vi "GCode Parser - SoftMotion Example.vi"() -> ()   [LabVIEW 2014]
uses:
  Typedefs/Motion Parameters.ctl
  <vilib>/Motion/Express/_s/nimc.fb.straightLineMove.blendMode.ctl
  GCode Parser/GCode Command Cluster.ctl
  <vilib>/Motion/Express/_s/nimc.ex.clearFaults.clearFaults.axis.vi
  <vilib>/Motion/Express/_s/nimc.ex.power.power.axis.vi
  <vilib>/Motion/Express/_s/nimc.ex.resetPosition.resetPosition.axis.vi
  <vilib>/Motion/Express/_s/nimc.ex.straightLineMove.startStraightLineMove.coordinate.modeAbsolute.blendEnable.1.vi
  <vilib>/Motion/Express/_s/nimc.ex.arcMove.startArcMove.coordinate.modeCircular.blendEnable.1.vi
  <vilib>/Motion/Express/_s/nimc.ex.stopMove.stop.coordinate.modeDecelerate.vi
  <vilib>/Motion/Express/_s/nimc.ex.read.readTrajectoryData.coordinate.vi
  <vilib>/Motion/Express/_s/nimc.ex.read.readExecutionData.axis.vi
  <vilib>/Motion/BlockNode/FB.NIMotion.xnode
  <vilib>/Motion/Express/_s/nimc.fb.arcMove.blendMode.ctl
panel:
  out "Current GCode Command":T1
  in  "Motion Parameters":T2={"timeout"=-1.0, "acceleration"=10000.0, "deceleration"=10000.0, "accel. jerk"=100000.0, "decel. jerk"=100000.0, "blend mode"=10551334, "blend delay"=-1.0, "smoothing"=0.5, "last blend"=FALSE} {"blend mode" items=["At Profile Complete"=10551335, "At Deceleration"=10551334, "After Delay"=10551336]}
  in  "G0 Velocity":dbl=20.0
  in  "Position Scale":dbl=1.0
  in  "Velocity Scale":dbl=1.0
  out "Global Stop":bool
  out "text":string
  in  "Quit":bool
  out "Iterations":i32
  out "Command Array":T1[](array[typedef])
  out "error out":errorcluster
  out "Position Plot":cluster{dbl[], dbl[]}(graph)
  out "Axis Positions":T4(graph)
  out "Axis Velocities":T5(graph)
  in  "start index":i32
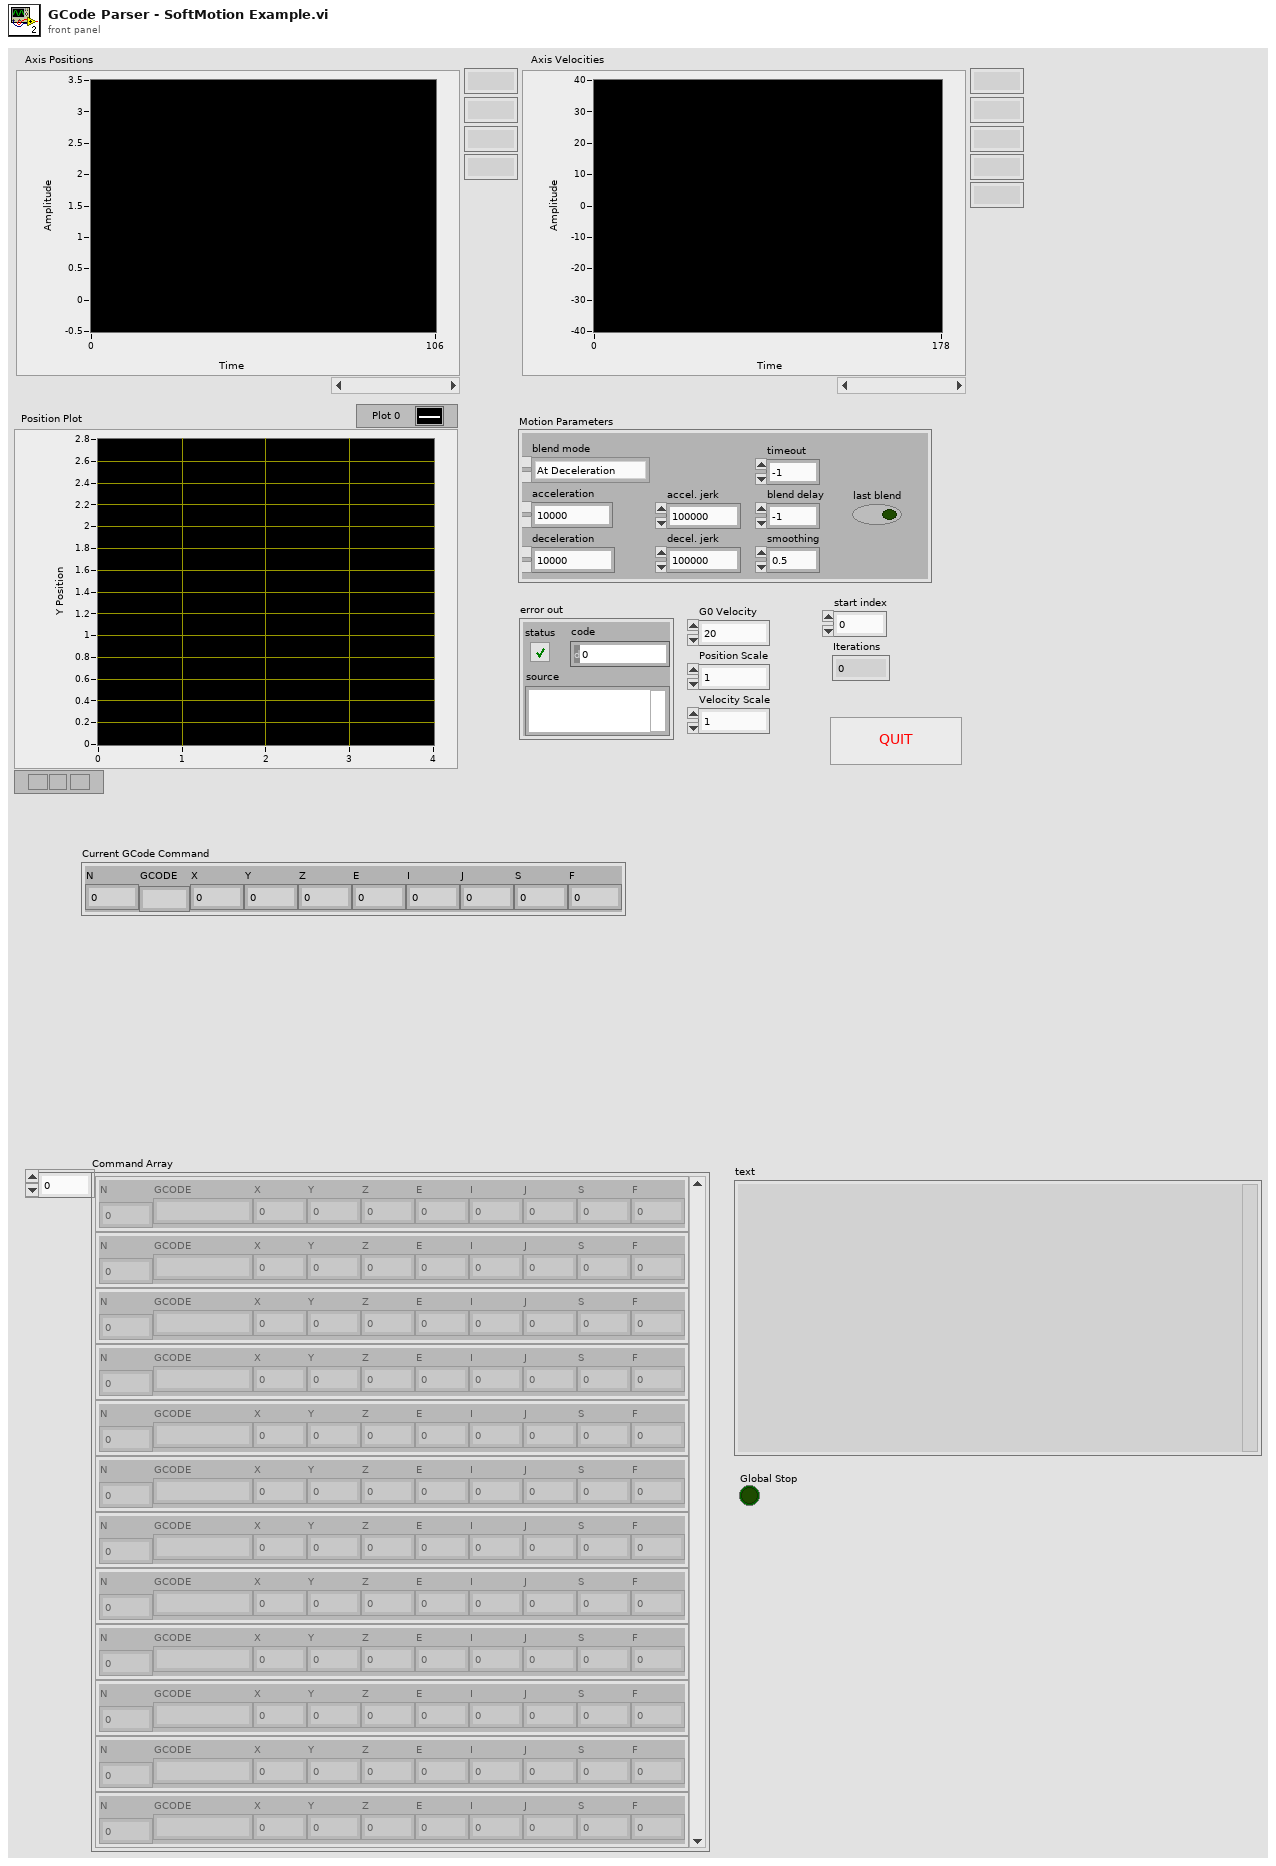
[diagram p1: front panel]
types:
  T1 = typedef "GCode Command Cluster.ctl" = cluster{"N":dbl, "GCODE":string, "X":dbl, "Y":dbl, "Z":dbl, "E":dbl, "I":dbl, "J":dbl, "S":dbl, "F":dbl}
  T2 = typedef "Motion Parameters.ctl" = cluster{"timeout":dbl, "acceleration":dbl, "deceleration":dbl, "accel. jerk":dbl, "decel. jerk":dbl, "blend mode":T3, "blend delay":dbl, "smoothing":dbl, "last blend":bool}
  T3 = typedef "nimc.fb.straightLineMove.blendMode.ctl" = i32
  T4 = cluster{"commanded pos.[] out[0]":dbl, "commanded pos.[] out[1]":dbl, "commanded pos.[] out[2]":dbl, "commanded pos.[] out[3]":dbl}
  T5 = cluster{"commanded vel.":dbl, "velocity":dbl, "velocity":dbl, "velocity":dbl, "velocity":dbl}
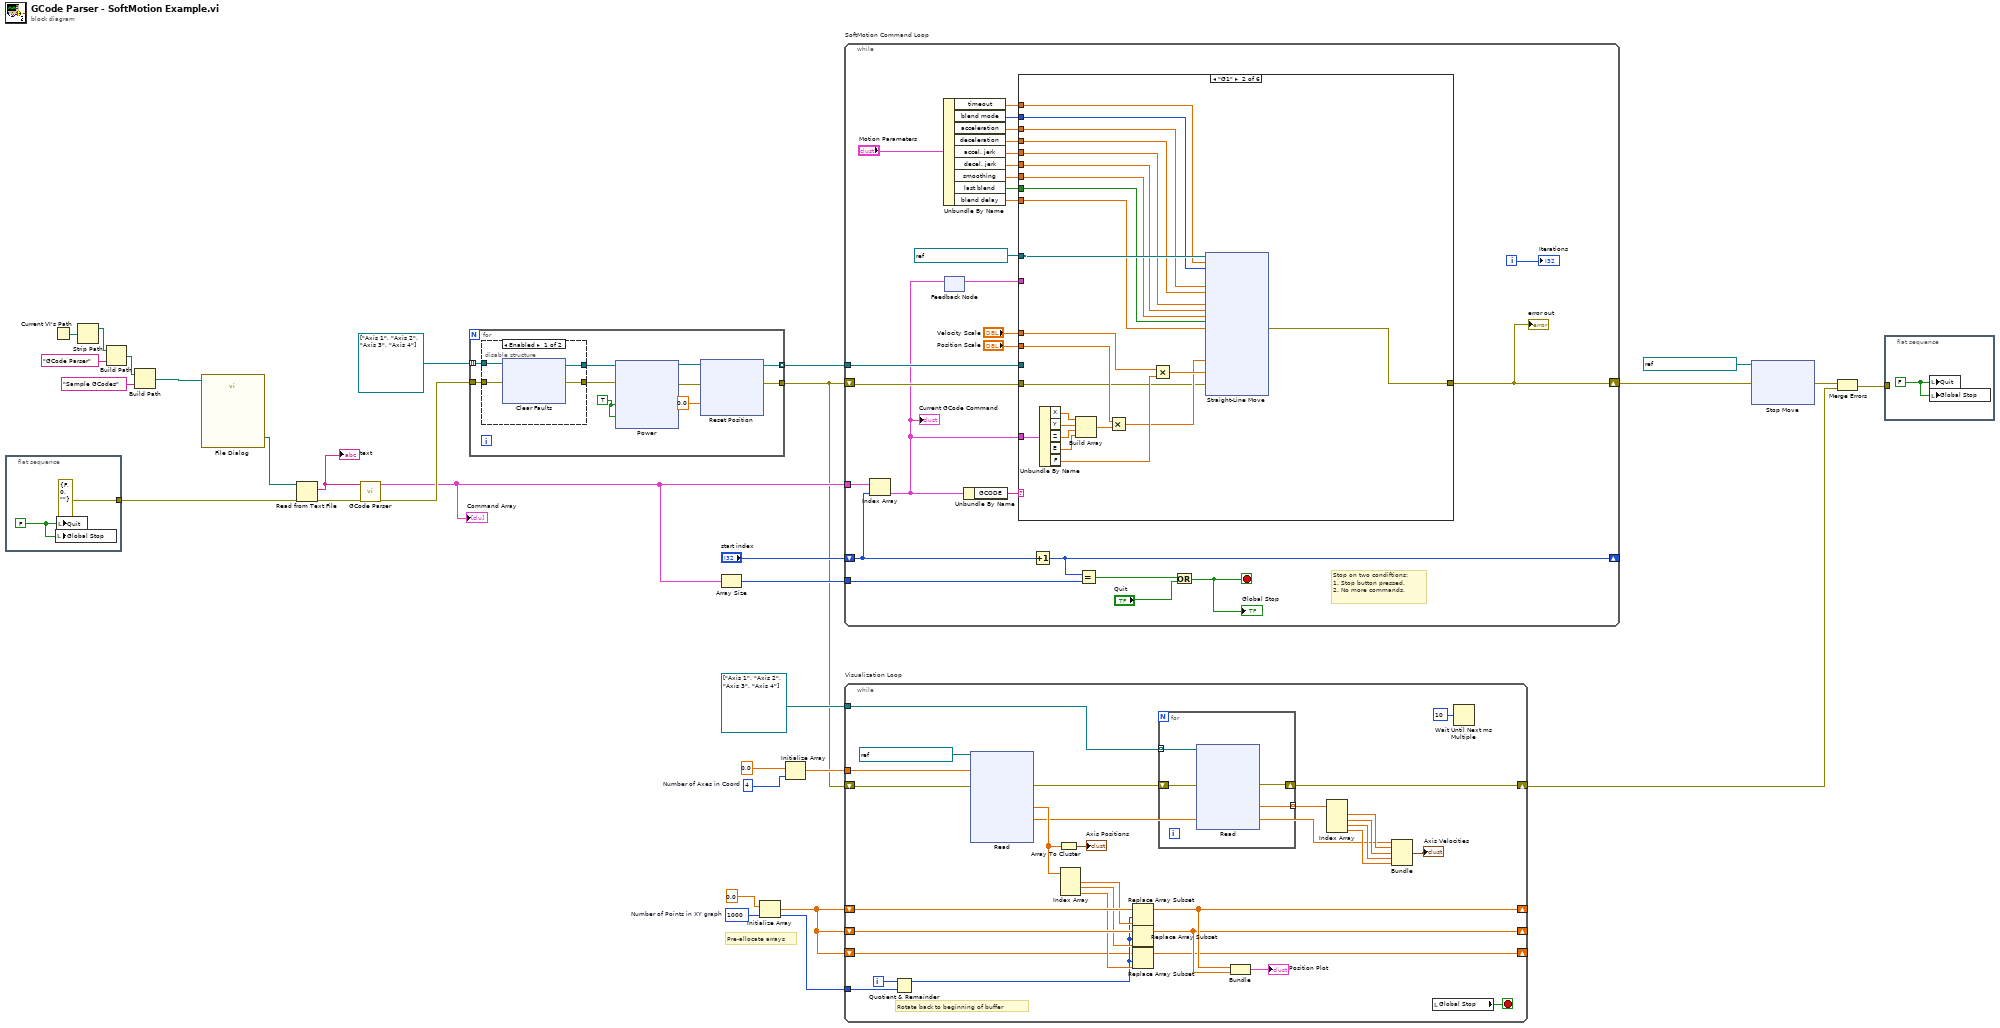
[diagram p0: block diagram]
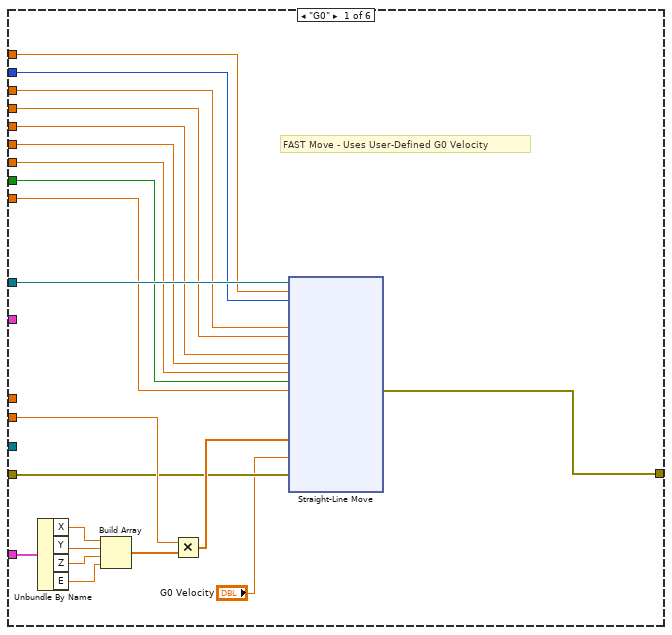
[diagram p2: hidden frame]
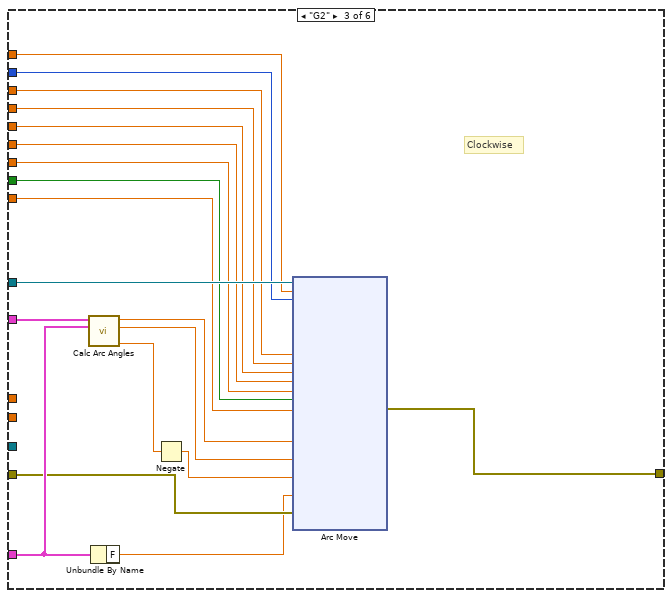
[diagram p3: hidden frame]
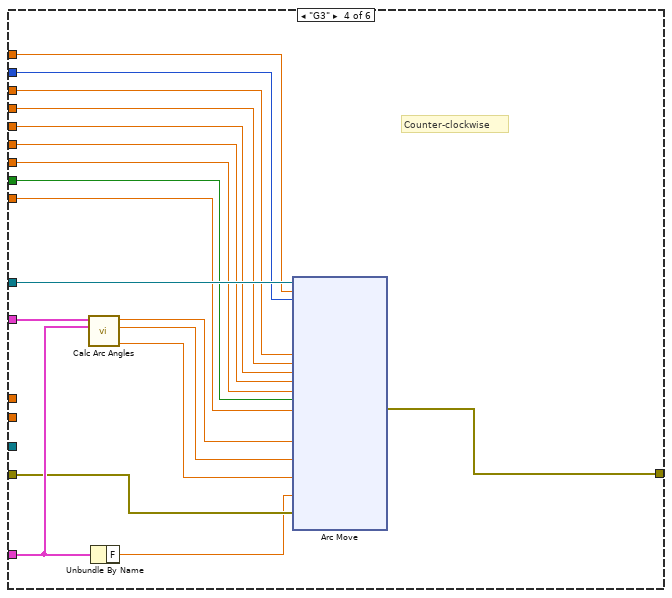
[diagram p4: hidden frame]
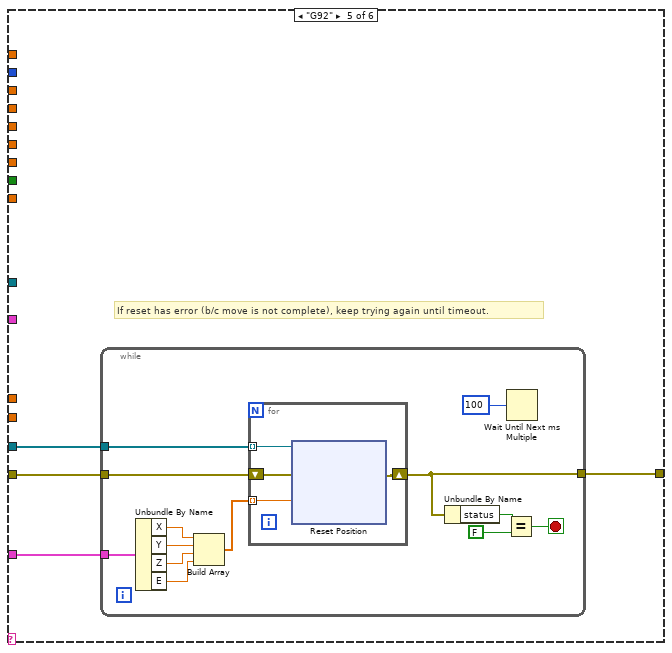
[diagram p5: hidden frame]
diagram:
  w25 = 1000  # Number of Points in XY graph
  w27 = 4  # Number of Axes in Coord
  # "Pre-allocate arrays"
  n1 = flat-sequence {
    tunnel: [errorcluster {"status"=FALSE, "code"=0, "source"=""} ("error out")] -> w20
    frame #0 {
      w30 = FALSE ("Example Done")
      n2 = local write "Global Stop"(w30) -> ()
      n3 = local write "Quit"(w30) -> ()
    }
  }
  n4 = Current VI's Path() -> (path=w7:path)
  n5 = Strip Path(path=w7) -> (stripped path=w6:path)  [unwired: 1 out]
  n6 = Build Path(base path=w6, name or relative path="GCode Parser") -> (appended path=w2:path)
  n7 = Build Path(base path=w2, name or relative path="Sample GCodes") -> (appended path=w1:path)
  n8 = call "File Dialog"("start path"=w1) -> ("selected path"=w4:path)  [unwired: 11 in, 3 out]
  n9 = Read from Text File(file (use dialog)=w4, error in=w20) -> (text=w22:string, error out=w21:errorcluster)  [unwired: 2 in, 2 out]
  "text" <- w22
  n10 = call "GCode Parser.vi"("error in (no error)"=w21, "String in"=w22) -> ("error out"=w19:errorcluster, "Command Array"=w15:T1[])  [unwired: 8 in]
  "Command Array" <- w15
  n11 = for {
    tunnel: refnum<k21>[] ["Axis 1", "Axis 2", "Axis 3", "Axis 4"] -> [w41] mode=indexing
    tunnel: w19 -> [w40]
    tunnel: [w39] -> w12
    tunnel: [w32] -> w16 mode=indexing
    w34 = TRUE ("enable axis")
    n12 = disable-structure shown="Enabled" {
      disable-tunnel: w41 -> [w45 w51]
      disable-tunnel: w40 -> [w44 w50]
      disable-tunnel: [w43 w51] -> w37
      disable-tunnel: [w42 w50] -> w35
      frame Enabled {
        n13 = xnode ("Clear Faults")("resource"=w45, "error in"=w44) -> ("resource out"=w43:refnum<k21>, "error out"=w42:errorcluster)
      }
      frame Disabled {
      }
    }
    n14 = xnode ("Power")("enable axis"=w34, "enable drive"=w34, "resource"=w37, "error in"=w35) -> ("resource out"=w36:refnum<k21>, "error out"=w33:errorcluster)
    n15 = xnode ("Reset Position")("position"=0.0, "resource"=w36, "error in"=w33) -> ("resource out"=w32:refnum<k21>, "error out"=w39:errorcluster)
  }
  n16 = Array Size(array=w15) -> (size(s)=w14:i32)
  n17 = Initialize Array(0.0 ("element"), w25) -> (w24:dbl[])
  n18 = Initialize Array(0.0 ("element"), w27) -> (w23:dbl[])
  n19 = while "SoftMotion Command Loop" {
    tunnel: w15 -> [w86]
    shift-right: [w83] -> _
    shift-left: "start index" -> [w85]
    shift-right: [w90] -> w9
    shift-left: w12 -> [w89]
    tunnel: w16 -> [w88]
    tunnel: w14 -> [w84]
    i -> [w87]
    stop <- w81 stop-if-true
    # "Stop on two condiftions:\n1. Stop button pressed.\n2. No more commands."
    n20 = Index Array(array=w86, index=w85) -> (element=w68:T1)
    "Current GCode Command" <- w68
    n21 = Unbundle By Name("Motion Parameters") -> ("timeout"=w77:dbl, "blend mode"=w76:T3, "acceleration"=w75:dbl, "deceleration"=w74:dbl, "accel. jerk"=w73:dbl, "decel. jerk"=w72:dbl, "smoothing"=w70:dbl, "last blend"=w71:bool, "blend delay"=w69:dbl)
    n22 = feedback-in #1(w68) -> ()
    n23 = feedback #1() -> (w67:T1)  [unwired: 1 in]
    n24 = Unbundle By Name(w68) -> ("GCODE"=w93:string)
    n25 = case shown="\"G1\"" w93 {
      tunnel: refnum<k21> "Coordinate Space 1" ("Motion Resource") -> [w106 w147 w196 w236 _ _]
      tunnel: [w114 w157 w186 w226 w259 w285] -> w90
      tunnel: "Velocity Scale" -> [_ w135 _ _ _ _]
      tunnel: w68 -> [w109 w151 w193 w233 w260 _]
      tunnel: "Position Scale" -> [w107 w148 _ _ _ _]
      tunnel: w89 -> [w104 w145 w187 w227 w261 w285]
      tunnel: w77 -> [w103 w144 w192 w232 _ _]
      tunnel: w76 -> [w102 w143 w178 w220 _ _]
      tunnel: w75 -> [w101 w142 w191 w231 _ _]
      tunnel: w74 -> [w100 w141 w190 w230 _ _]
      tunnel: w73 -> [w99 w140 w189 w229 _ _]
      tunnel: w72 -> [w98 w139 w188 w228 _ _]
      tunnel: w70 -> [w97 w138 w179 w221 _ _]
      tunnel: w71 -> [w96 w137 w180 w222 _ _]
      tunnel: w69 -> [w95 w136 w181 w223 _ _]
      tunnel: w88 -> [_ _ _ _ w262 _]
      tunnel: w67 -> [_ _ w195 w235 _ _]
      frame "G0" {
        # "FAST Move - Uses User-Defined G0 Velocity"
        n26 = Unbundle By Name(w109) -> ("X"=w113:dbl, "Y"=w112:dbl, "Z"=w111:dbl, "E"=w110:dbl)
        n27 = Build Array(w113, w112, w111, w110) -> (w108:dbl[])
        n28 = Multiply(x=w107, y=w108) -> (x*y=w105:dbl[])
        n29 = xnode ("Straight-Line Move")("position[]"=w105, "velocity"="G0 Velocity", "error in"=w104, "resource"=w106, "timeout"=w103, "blend mode"=w102, "acceleration"=w101, "deceleration"=w100, "accel. jerk"=w99, "decel. jerk"=w98, "smoothing"=w97, "last blend"=w96, "blend delay"=w95) -> ("error out"=w114:errorcluster)  [unwired: 2 out]
      }
      frame "G1" {
        n30 = Unbundle By Name(w151) -> ("X"=w156:dbl, "Y"=w155:dbl, "Z"=w154:dbl, "E"=w153:dbl, "F"=w152:dbl)
        n31 = Build Array(w156, w155, w154, w153) -> (w149:dbl[])
        n32 = Multiply(x=w148, y=w149) -> (x*y=w146:dbl[])
        n33 = Multiply(x=w135, y=w152) -> (x*y=w150:dbl)
        n34 = xnode ("Straight-Line Move")("position[]"=w146, "velocity"=w150, "error in"=w145, "resource"=w147, "timeout"=w144, "blend mode"=w143, "acceleration"=w142, "deceleration"=w141, "accel. jerk"=w140, "decel. jerk"=w139, "smoothing"=w138, "last blend"=w137, "blend delay"=w136) -> ("error out"=w157:errorcluster)  [unwired: 2 out]
      }
      frame "G2" {
        # "Clockwise"
        n35 = call "Calc Arc Angles.vi"("Arc CMD"=w193, "Initial CMD"=w195) -> ("travel angle out"=w184:dbl, "start angle (tangent)"=w183:dbl, "R"=w194:dbl)  [unwired: 7 in]
        n36 = Unbundle By Name(w193) -> ("F"=w182:dbl)
        n37 = Negate(x=w184) -> (-x=w185:dbl)
        n38 = xnode ("Arc Move")("radius"=w194, "start angle"=w183, "travel angle"=w185, "velocity"=w182, "error in"=w187, "resource"=w196, "timeout"=w192, "blend mode"=w178, "acceleration"=w191, "deceleration"=w190, "accel. jerk"=w189, "decel. jerk"=w188, "smoothing"=w179, "last blend"=w180, "blend delay"=w181) -> ("error out"=w186:errorcluster)  [unwired: 2 out]
      }
      frame "G3" {
        # "Counter-clockwise"
        n39 = call "Calc Arc Angles.vi"("Arc CMD"=w233, "Initial CMD"=w235) -> ("travel angle out"=w219:dbl, "start angle (tangent)"=w225:dbl, "R"=w234:dbl)  [unwired: 7 in]
        n40 = Unbundle By Name(w233) -> ("F"=w224:dbl)
        n41 = xnode ("Arc Move")("radius"=w234, "start angle"=w225, "travel angle"=w219, "velocity"=w224, "error in"=w227, "resource"=w236, "timeout"=w232, "blend mode"=w220, "acceleration"=w231, "deceleration"=w230, "accel. jerk"=w229, "decel. jerk"=w228, "smoothing"=w221, "last blend"=w222, "blend delay"=w223) -> ("error out"=w226:errorcluster)  [unwired: 2 out]
      }
      frame "G92" {
        # "If reset has error (b/c move is not complete), keep trying again until timeout."
        n42 = while {
          tunnel: [w272] -> w259
          tunnel: w262 -> [w270]
          tunnel: w261 -> [w269]
          tunnel: w260 -> [w264]
          stop <- w271 stop-if-true
          n43 = Unbundle By Name(w264) -> ("X"=w268:dbl, "Y"=w267:dbl, "Z"=w266:dbl, "E"=w265:dbl)
          n44 = Build Array(w268, w267, w266, w265) -> (w263:dbl[])
          n45 = for {
            tunnel: w270 -> [w278] mode=indexing
            shift-right: [w279] -> w272
            shift-left: w269 -> [w277]
            tunnel: w263 -> [w276] mode=indexing
            n46 = xnode ("Reset Position")("position"=w276, "resource"=w278, "error in"=w277) -> ("error out"=w279:errorcluster)  [unwired: 1 out]
          }
          n47 = Unbundle By Name(w272) -> ("status"=w274:bool)
          n48 = Equal?(x=w274, y=FALSE) -> (x = y?=w271:bool)
          n49 = Wait Until Next ms Multiple(millisecond multiple=u32 100) -> ()  [unwired: 1 out]
        }
      }
      frame Default {
        # "Empty case for all other codes."
      }
    }
    "error out" <- w90
    n50 = Increment(x=w85) -> (x+1=w83:i32)
    n51 = Equal?(x=w83, y=w84) -> (x = y?=w82:bool)
    n52 = Or(x=w82, y="Quit") -> (x .or. y?=w81:bool)
    "Global Stop" <- w81
    "Iterations" <- w87
  }
  n53 = while "Visualization Loop" {
    shift-right: [w304] -> _
    shift-left: w24 -> [w314]
    shift-right: [w286] -> w11
    shift-left: w12 -> [w294]
    shift-right: [w303] -> _
    shift-left: w24 -> [w312]
    tunnel: w25 -> [w309]
    shift-right: [w302] -> _
    shift-left: w24 -> [w305]
    tunnel: w23 -> [w291]
    tunnel: refnum<k21>[] ["Axis 1", "Axis 2", "Axis 3", "Axis 4"] -> [w300]
    i -> [w308]
    stop <- w288 stop-if-true
    # "Rotate back to beginning of buffer"
    n54 = Quotient & Remainder(x=w308, y=w309) -> (x-y*floor(x/y)=w306:i32)  [unwired: 1 out]
    n55 = xnode ("Read")("resource"=refnum<k21> "Coordinate Space 1" ("Motion Resource"), "commanded pos.[]"=w291, "error in"=w294) -> ("commanded pos.[] out"=w292:dbl[], "commanded vel."=w289:dbl, "error out"=w293:errorcluster)  [unwired: 3 out]
    n56 = Array To Cluster(array=w292) -> (cluster=→"Axis Positions":T4)
    n57 = Index Array(array=w292) -> (element #1=w313:dbl, element #2=w311:dbl, element #3=w307:dbl)  [unwired: 3 in]
    n58 = Replace Array Subset(array=w314, new element=w313, index=w306) -> (w304:dbl[])
    n59 = Replace Array Subset(array=w312, new element=w311, index=w306) -> (w303:dbl[])
    n60 = Replace Array Subset(array=w305, new element=w307, index=w306) -> (w302:dbl[])
    n61 = for {
      tunnel: w300 -> [w328] mode=indexing
      tunnel: [w327] -> w299 mode=indexing
      shift-right: [w325] -> w286
      shift-left: w293 -> [w326]
      n62 = xnode ("Read")("resource"=w328, "error in"=w326) -> ("velocity"=w327:dbl, "error out"=w325:errorcluster)  [unwired: 5 out]
    }
    n63 = Bundle(w304, w303) -> (→"Position Plot":cluster{dbl[], dbl[]})  [unwired: 1 in]
    n64 = Index Array(array=w299) -> (element #1=w298:dbl, element #2=w297:dbl, element #3=w296:dbl, element #4=w290:dbl)  [unwired: 4 in]
    n65 = Bundle("commanded vel."=w289, "velocity"=w298, "velocity"=w297, "velocity"=w296, "velocity"=w290) -> (→"Axis Velocities":T5)  [unwired: 1 in]
    n66 = local read "Global Stop"() -> (w288:bool)
    n67 = Wait Until Next ms Multiple(millisecond multiple=u32 10) -> ()  [unwired: 1 out]
  }
  n68 = xnode ("Stop Move")("resource"=refnum<k21> "Coordinate Space 1" ("coordinate"), "error in"=w9) -> ("error out"=w8:errorcluster)  [unwired: 1 in, 2 out]
  n69 = Merge Errors(w8, w11) -> (w13:errorcluster)
  n70 = flat-sequence {
    tunnel: w13 -> [_]
    frame #0 {
      w338 = FALSE ("Example Done")
      n71 = local write "Quit"(w338) -> ()
      n72 = local write "Global Stop"(w338) -> ()
    }
  }
